vi "Stop Core.vi"(10 "final error code":i32 caption="最终错误代码", 11 "上位机代理者 in":refnum<class "服务器.lvclass"> caption="操作者输入") -> (3 "上位机代理者 out":refnum<class "服务器.lvclass"> caption="操作者输出")   [LabVIEW 2015, in "服务器.lvlib" / "服务器.lvclass"]
doc: "(<B>Filename</B>: Actor Framework.lvlib:Actor.lvclass:Stop Core.vi)\n\nDefines what the actor does before it stops. Use the <B>final error code</B> input to determine whether the actor shut down in response to an error.\n\nBy default, this method does nothing. A descendant class may override it to define behavior, such as shutting down any processes the actor initiated in its override of the Actor Core method."
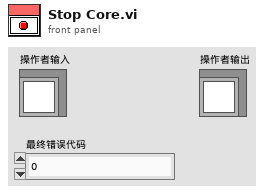
[diagram p1: front panel]
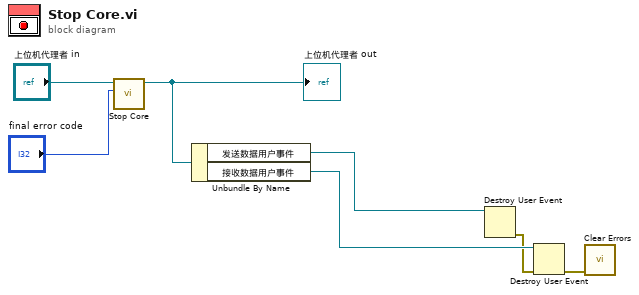
[diagram p0: block diagram]
diagram:
  n1 = call-parent "Stop Core.vi"("final error code"="final error code", "前面板控制 in"="上位机代理者 in") -> ("前面板控制 out"=w1:refnum<class "服务器.lvclass">)  [unwired: 9 in]
  "上位机代理者 out" <- w1
  n2 = Unbundle By Name(w1) -> ("发送数据用户事件"=w5:refnum<user-event>, "接收数据用户事件"=w4:refnum<user-event>)
  n3 = Destroy User Event(user event=w5) -> (error out=w3:errorcluster)  [unwired: 1 in]
  n4 = Destroy User Event(user event=w4, error in=w3) -> (error out=w2:errorcluster)
  n5 = call <vilib>:"Clear Errors.vi"("error in (no error)"=w2) -> ()  [unwired: 5 in, 2 out]
